vi "Initialize_loop.vi"(11 "error in (no error)":errorcluster) -> (3 "error out":errorcluster)   [LabVIEW 2016]
uses:
  <vilib>/myRIO/Instrument Drivers/Onboard IO/DIO/typedefs/DIO Reference.ctl
  <vilib>/myRIO/Common/Instrument Driver Framework/Utilities/typedefs/myRIO Generic Hardware Reference.ctl
  <vilib>/myRIO/Common/Instrument Driver Framework/Utilities/typedefs/Hardware Version Enum.ctl
  <vilib>/myRIO/Common/Instrument Driver Framework/Utilities/typedefs/myRIO v1.0 Reference.ctl
  <vilib>/myRIO/Common/Instrument Driver Framework/Utilities/typedefs/Generic FPGA Reference.ctl
  <vilib>/myRIO/Common/Instrument Driver Framework/myRIO v1.0/DIO/typedefs/DIO Channels List.ctl
  <vilib>/myRIO/Common/Instrument Driver Framework/myRIO v1.0/DIO/typedefs/DIO Channels Enum.ctl
  <vilib>/userdefined/High Color/nirio_resource_hc.ctl
  <vilib>/myRIO/Instrument Drivers/Onboard IO/SPI/typedefs/SPI User Configuration.ctl
  <vilib>/myRIO/Common/Instrument Driver Framework/myRIO v1.0/SPI/typedefs/SPI Clock Phase.ctl
  <vilib>/myRIO/Common/Instrument Driver Framework/myRIO v1.0/SPI/typedefs/SPI Clock Polarity.ctl
  <vilib>/myRIO/Common/Instrument Driver Framework/myRIO v1.0/SPI/typedefs/SPI Data Direction.ctl
  <vilib>/myRIO/Common/Instrument Driver Framework/myRIO v1.0/SPI/typedefs/SPI Frame Length.ctl
  <vilib>/myRIO/Instrument Drivers/Onboard IO/SPI/typedefs/SPI Reference.ctl
  <vilib>/myRIO/Common/Instrument Driver Framework/myRIO v1.0/SPI/typedefs/SPI Channels Enum.ctl
  <vilib>/myRIO/Instrument Drivers/Onboard IO/SPI/typedefs/SPI Configuration.ctl
  <vilib>/myRIO/Common/Instrument Driver Framework/Utilities/vis/Is FPGA Ref Available.vi
  <vilib>/myRIO/Common/Instrument Driver Framework/roboRIO v1.0/DIO/vis/roboRIO v1.0 Open DIO.vi
  <vilib>/myRIO/Instrument Drivers/Onboard IO/DIO/vis/Write.vi
  <vilib>/myRIO/Common/Instrument Driver Framework/roboRIO v1.0/SPI/vis/roboRIO v1.0 Open SPI.vi
  <vilib>/myRIO/Instrument Drivers/Onboard IO/SPI/vis/Configure.vi
  <vilib>/myRIO/Instrument Drivers/Onboard IO/SPI/vis/Write Read.vi
  <vilib>/myRIO/Common/Instrument Driver Framework/Utilities/vis/Validate Channels.vi
  <vilib>/myRIO/Common/Instrument Driver Framework/roboRIO v1.0/DIO/vis/roboRIO v1.0 Reserve DIO.vi
  <vilib>/myRIO/Common/Instrument Driver Framework/roboRIO v1.0/SPI/vis/roboRIO v1.0 Reserve SPI.vi
  <vilib>/myRIO/Common/Instrument Driver Framework/roboRIO v1.0/DIO/vis/roboRIO v1.0 Build MUX Configuration DIO.vi
  <vilib>/myRIO/Common/Instrument Driver Framework/roboRIO v1.0/Resource Manager/vis/roboRIO v1.0 Reserve Channel List.vi
  <vilib>/myRIO/Common/Instrument Driver Framework/roboRIO v1.0/SPI/vis/roboRIO v1.0 Build MUX Configuration SPI.vi
  <vilib>/myRIO/Common/Instrument Driver Framework/roboRIO v1.0/Resource Manager/vis/roboRIO v1.0 Create Configuration List.vi
  <vilib>/myRIO/Common/Instrument Driver Framework/roboRIO v1.0/Resource Manager/vis/roboRIO v1.0 Reserve Channel.vi
  <vilib>/myRIO/Common/Instrument Driver Framework/roboRIO v1.0/Resource Manager/vis/roboRIO v1.0 Unreserve Channel.vi
  <vilib>/myRIO/Common/Instrument Driver Framework/myRIO v1.0/Resource Manager/vis/myRIO v1.0 Create Configuration List.vi
  <vilib>/myRIO/Common/Instrument Driver Framework/roboRIO v1.0/Resource Manager/vis/roboRIO v1.0 Build Mutex Name.vi
  <vilib>/Utility/VariantDataType/GetNumericInfo.vi
  <vilib>/Utility/error.llb/Error Cluster From Error Code.vi
  <vilib>/myRIO/Common/Instrument Driver Framework/roboRIO v1.0/roboRIO v1.0 Open.vi
  <vilib>/myRIO/Common/Instrument Driver Framework/Utilities/vis/IO Manager.vi
  <vilib>/myRIO/Common/Instrument Driver Framework/Utilities/vis/Configuration Manager.vi
  <vilib>/myRIO/Common/Instrument Driver Framework/roboRIO v1.0/Resource Manager/vis/roboRIO v1.0 Configure IO.vi
  <vilib>/myRIO/Common/Instrument Driver Framework/myRIO v1.0/myRIO v1.0 Close.vi
  <vilib>/myRIO/Common/Instrument Driver Framework/roboRIO v1.0/DIO/vis/roboRIO v1.0 Write DIO.vi
  <vilib>/myRIO/Common/Instrument Driver Framework/roboRIO v1.0/SPI/vis/roboRIO v1.0 Configure SPI.vi
  <vilib>/myRIO/Common/Instrument Driver Framework/roboRIO v1.0/SPI/vis/roboRIO v1.0 Write Read SPI.vi
  <vilib>/myRIO/Express VI/Onboard IO/DO/DO Express VI.xnode
  <vilib>/myRIO/Instrument Drivers/Onboard IO/DIO/vis/myRIO DIO Open.xnode
  <vilib>/myRIO/Express VI/Onboard IO/SPI/SPI Express VI.xnode
  <vilib>/myRIO/Instrument Drivers/Onboard IO/SPI/vis/myRIO SPI Open.xnode
  <vilib>/myRIO/Instrument Drivers/Onboard IO/DIO/DIO.lvlib
  <vilib>/myRIO/Instrument Drivers/Onboard IO/SPI/SPI.lvlib
panel:
  out "Frames Read":u16[](array[numeric])
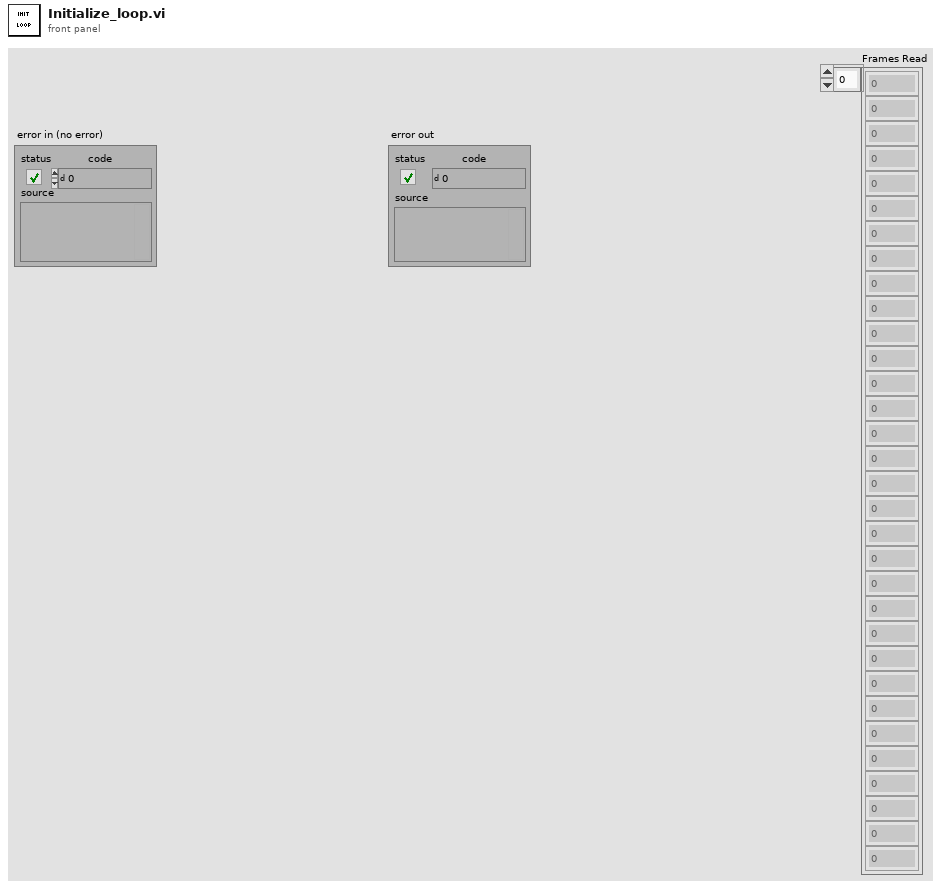
[diagram p1: front panel]
types:
  T1 = typedef "DIO.lvlib/DIO Reference.ctl" = cluster{"myRIO Reference":T2, "DIO Channels List":T6}
  T2 = typedef "myRIO Generic Hardware Reference.ctl" = cluster{"myRIO Model":T3, "myRIO Hardware Reference":T4}
  T3 = typedef "Hardware Version Enum.ctl" = enum16{"Unknown", "myRIO-1900", "myRIO-1950", "roboRIO", "NI ELVIS RIO CM"}
  T4 = typedef "myRIO v1.0 Reference.ctl" = cluster{"Generic FPGA Reference":T5, "Allow multiple opens":bool}
  T5 = typedef "Generic FPGA Reference.ctl" = refnum<k20>
  T6 = typedef "DIO Channels List.ctl" = T7[]
  T7 = typedef "DIO Channels Enum.ctl" = enum16{"Not Connected", "C/DIO0", "C/DIO1", "C/DIO2", "C/DIO3", "C/DIO4", "C/DIO5", "C/DIO6", "C/DIO7", "A/DIO0", "A/DIO1", "A/DIO2", "A/DIO3", "A/DIO4", "A/DIO5", "A/DIO6", "A/DIO7", "A/DIO8", "A/DIO9", "A/DIO10", "A/DIO11", "A/DIO12", "A/DIO13", "A/DIO14", "A/DIO15", "B/DIO0", "B/DIO1", "B/DIO2", "B/DIO3", "B/DIO4", "B/DIO5", "B/DIO6", "B/DIO7", "B/DIO8", "B/DIO9", "B/DIO10", "B/DIO11", "B/DIO12", "B/DIO13", "B/DIO14", "B/DIO15", "LED0", "LED1", "LED2", "LED3", "Button0", "DIO/DIO0", "DIO/DIO1", "DIO/DIO2", "DIO/DIO3", "DIO/DIO4", "DIO/DIO5", "DIO/DIO6", "DIO/DIO7", "DIO/DIO8", "DIO/DIO9", "SPI/CS0", "SPI/CS1", "SPI/CS2", "SPI/CS3", "LED RADIO (Green)", "LED RADIO (Red)", "LED COMM (Green)", "LED COMM (Red)", "LED MODE (Green)", "LED MODE (Red)"}
  T8 = typedef "nirio_resource_hc.ctl" = tag
  T9 = typedef "SPI.lvlib/SPI Reference.ctl" = cluster{"myRIO Reference":T2, "SPI Channels Enum":T10, "SPI Configuration":T11}
  T10 = typedef "SPI Channels Enum.ctl" = enum16{"Not Connected", "A/SPI", "B/SPI", "SPI/SPI"}
  T11 = typedef "SPI.lvlib/SPI Configuration.ctl" = cluster{"Frequency [Hz]":dbl, "Clock Phase":T12, "Clock Polarity":T13, "Data Direction":T14, "Frame Length":T15}
  T12 = typedef "SPI Clock Phase.ctl" = enum8{"Leading", "Trailing"}
  T13 = typedef "SPI Clock Polarity.ctl" = enum8{"Low", "High"}
  T14 = typedef "SPI Data Direction.ctl" = enum8{"Most significant bit first", "Least significant bit first"}
  T15 = typedef "SPI Frame Length.ctl" = u8
  T16 = typedef "SPI.lvlib/SPI User Configuration.ctl" = cluster{"Frequency [Hz]":dbl, "Clock Phase":T12, "Clock Polarity":T13, "Data Direction":T14, "Frame Length":T15}
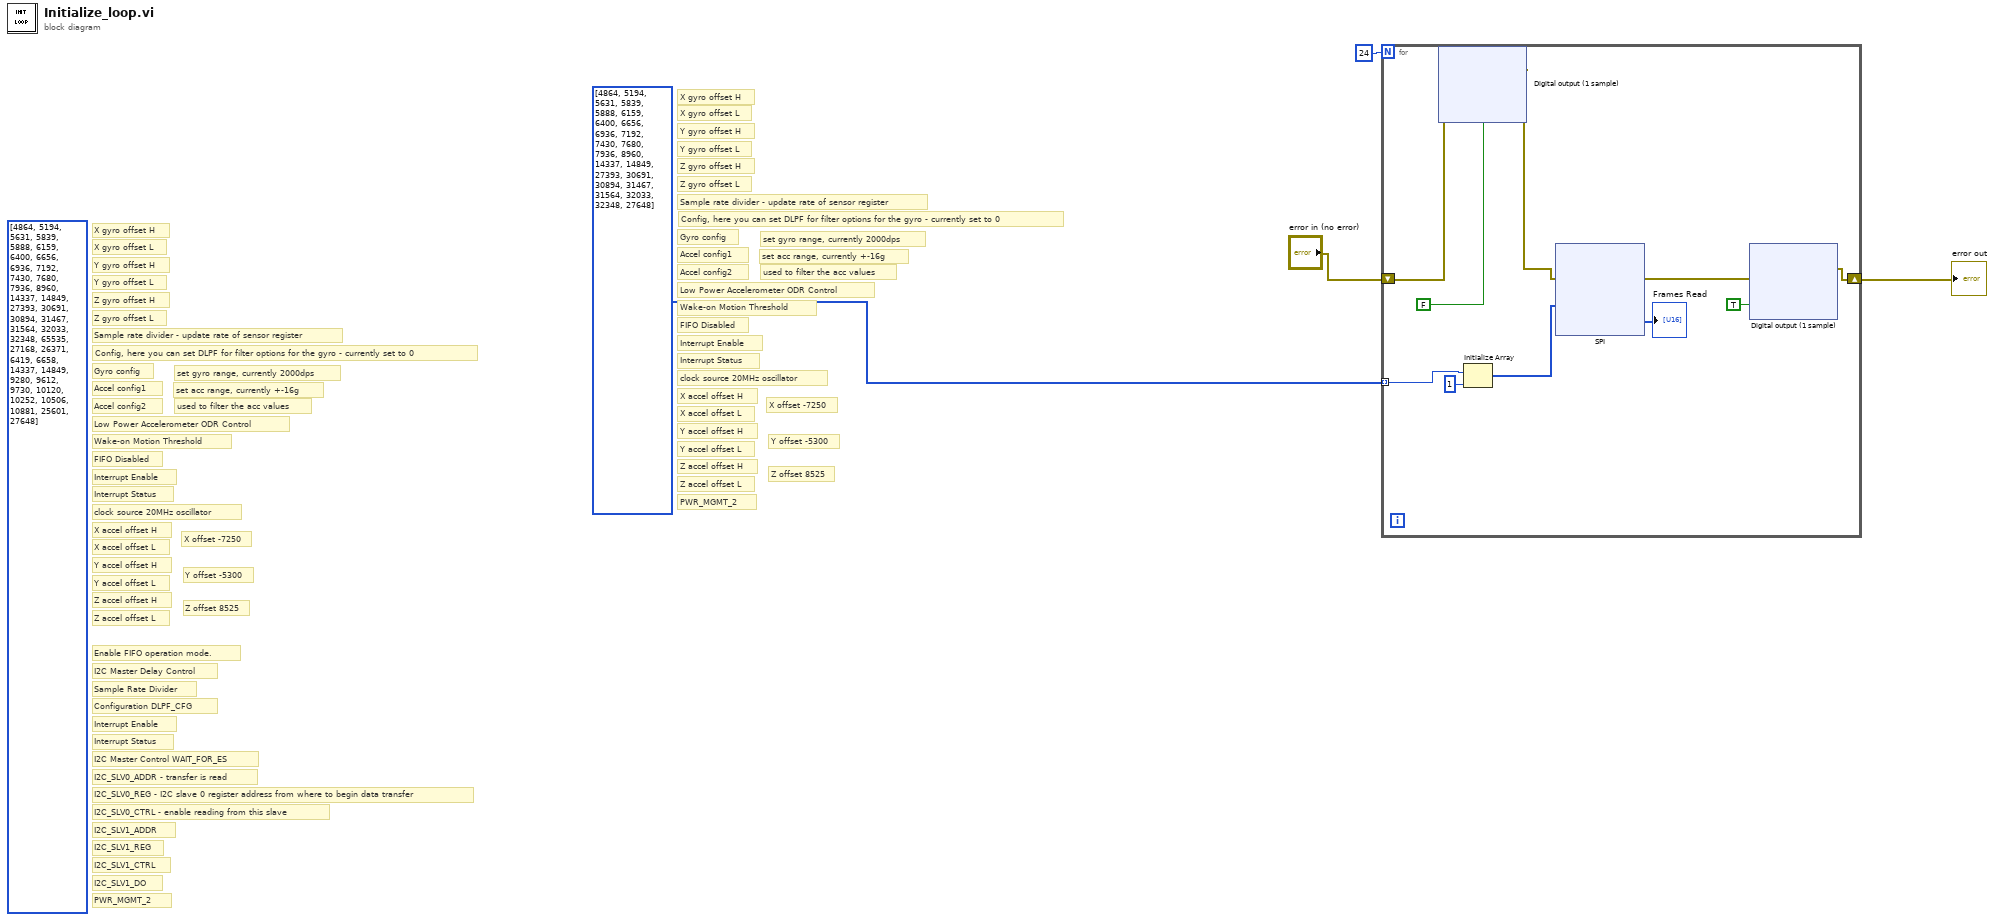
[diagram p0: block diagram]
diagram:
  (unwired) u16[] [4864, 5194, 5631, 5839, 5888, 6159, 6400, 6656, 6936, 7192, 7430, 7680, 7936, 8960, 14337, 14849, 27393, 30691, 30894, 31467, 31564, 32033, 32348, 65535, 27168, 26371, 6419, 6658, 14337, 14849, 9280, 9612, 9730, 10120, 10252, 10506, 10881, 25601, 27648]
  # "used to filter the acc values"
  # "PWR_MGMT_2"
  # "I2C_SLV1_DO"
  # "I2C_SLV1_CTRL"
  # "I2C_SLV1_REG"
  # "I2C_SLV1_ADDR"
  # "I2C_SLV0_CTRL - enable reading from this slave"
  # "I2C_SLV0_REG - I2C slave 0 register address from where to begin data transfer"
  # "I2C_SLV0_ADDR - transfer is read"
  # "I2C Master Control WAIT_FOR_ES"
  # "Interrupt Status"
  # "Interrupt Enable"
  # "Configuration DLPF_CFG"
  # "Sample Rate Divider"
  # "I2C Master Delay Control"
  # "Enable FIFO operation mode."
  # "clock source 20MHz oscillator"
  # "Interrupt Status"
  # "Interrupt Enable"
  # "FIFO Disabled"
  # "Wake-on Motion Threshold"
  # "Low Power Accelerometer ODR Control"
  # "Accel config2"
  # "Accel config1"
  # "Gyro config"
  # "Config, here you can set DLPF for filter options for the gyro - currently set to 0"
  # "Sample rate divider - update rate of sensor register"
  # "Z gyro offset L"
  # "Y gyro offset L"
  # "X gyro offset L"
  # "Y accel offset L"
  # "X accel offset L"
  # "Z gyro offset H"
  # "Y gyro offset H"
  # "X gyro offset H"
  # "Y accel offset H"
  # "X accel offset H"
  # "Z accel offset L"
  # "Z accel offset H"
  # "set acc range, currently +-16g"
  # "set gyro range, currently 2000dps"
  # "Z offset 8525"
  # "Y offset -5300"
  # "X offset -7250"
  # "used to filter the acc values"
  # "PWR_MGMT_2"
  # "clock source 20MHz oscillator"
  # "Interrupt Status"
  # "Interrupt Enable"
  # "FIFO Disabled"
  # "Wake-on Motion Threshold"
  # "Low Power Accelerometer ODR Control"
  # "Accel config2"
  # "Accel config1"
  # "Gyro config"
  # "Config, here you can set DLPF for filter options for the gyro - currently set to 0"
  # "Sample rate divider - update rate of sensor register"
  # "Z gyro offset L"
  # "Y gyro offset L"
  # "X gyro offset L"
  # "Y accel offset L"
  # "X accel offset L"
  # "Z gyro offset H"
  # "Y gyro offset H"
  # "X gyro offset H"
  # "Y accel offset H"
  # "X accel offset H"
  # "Z accel offset L"
  # "Z accel offset H"
  # "set acc range, currently +-16g"
  # "set gyro range, currently 2000dps"
  # "Z offset 8525"
  # "Y offset -5300"
  # "X offset -7250"
  n1 = for {
    N: 24 -> [_]
    tunnel: u16[] [4864, 5194, 5631, 5839, 5888, 6159, 6400, 6656, 6936, 7192, 7430, 7680, 7936, 8960, 14337, 14849, 27393, 30691, 30894, 31467, 31564, 32033, 32348, 27648] -> [w8] mode=indexing
    shift-right: [w6] -> w2
    shift-left: "error in (no error)" -> [w5]
    n2 = xnode "Digital output (1 sample)"("SPI/CS0 (Pin 2)"=FALSE ("A/DIO0 (Pin 11)"), "error in (no error)"=w5) -> ("error out"=w11:errorcluster)
    n3 = Initialize Array(w8, 1 ("dimension size")) -> (w7:u16[])
    n4 = xnode "SPI"("Frames to Write"=w7, "error in (no error)"=w11) -> ("Frames Read"=→"Frames Read":u16[], "error out"=w13:errorcluster)
    n5 = xnode "Digital output (1 sample)"("SPI/CS0 (Pin 2)"=TRUE ("A/DIO0 (Pin 11)"), "error in (no error)"=w13) -> ("error out"=w6:errorcluster)
  }
  "error out" <- w2
